vi "SortControlTerminals.vi"(10 "error in":errorcluster, 11 "ControlTerminals in":refnum<class "ControlTerminal.lvclass">[](array[class])) -> (2 "error out":errorcluster, 3 "ControlTerminals out":refnum<class "ControlTerminal.lvclass">[](array[class]))   [LabVIEW 2014, in "ControlTerminal.lvclass"]
uses:
  ControlTerminal.lvclass
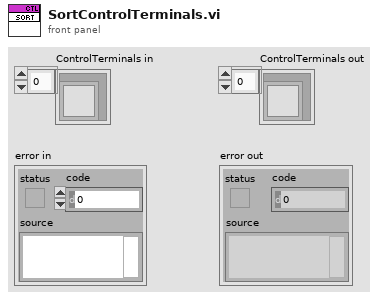
[diagram p1: front panel]
types:
  T1 = cluster{"terminal index":i32, "Control Terminal out":refnum<class "ControlTerminal.lvclass">}
  T2 = cluster{"terminal index":i32, "Control Terminal out":refnum<class "ControlTerminal.lvclass">}[]
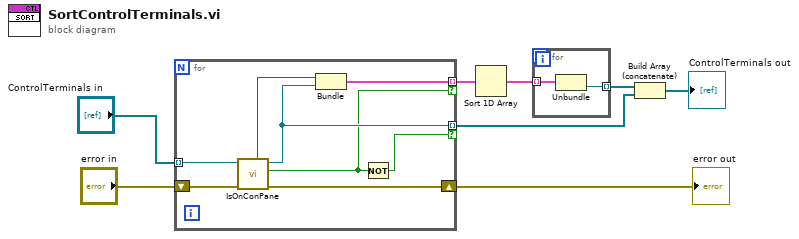
[diagram p0: block diagram]
diagram:
  n1 = for {
    tunnel: "ControlTerminals in" -> [w16] mode=indexing
    tunnel: [w13] -> w4 mode=indexing if=w15
    tunnel: [w12] -> w7 mode=indexing if=w11
    shift-right: [w9] -> w1
    shift-left: "error in" -> [w10]
    n2 = call "IsOnConPane.vi"("error in"=w10, "Control Terminal in"=w16) -> ("error out"=w9:errorcluster, "wired"=w11:bool, "Control Terminal out"=w13:refnum<class "ControlTerminal.lvclass">, "terminal index"=w14:i32)  [unwired: 4 in]
    n3 = Bundle("terminal index"=w14, "Control Terminal out"=w13) -> (w12:T1)  [unwired: 1 in]
    n4 = Not(x=w11) -> (.not. x?=w15:bool)
  }
  "error out" <- w1
  n5 = Sort 1D Array(array=w7) -> (sorted array=w6:T2)
  n6 = for {
    tunnel: w6 -> [w18] mode=indexing
    tunnel: [w17] -> w5 mode=indexing
    n7 = Unbundle(w18) -> ("Control Terminal out"=w17:refnum<class "ControlTerminal.lvclass">)  [unwired: 1 out]
  }
  n8 = Build Array (concatenate)(w5, w4) -> (→"ControlTerminals out":refnum<class "ControlTerminal.lvclass">[])
